vi "Write folder.vi"(8 "error in (no error)":errorcluster, 10 "folder":string="c:\\errorlog", 11 "SimpleErrorLogger in":refnum<class "SimpleErrorLogger.lvclass">) -> (0 "error out":errorcluster, 3 "SimpleErrorLogger out":refnum<class "SimpleErrorLogger.lvclass">)   [LabVIEW 2023, in "SimpleErrorLogger.lvlib" / "SimpleErrorLogger.lvclass"]
uses:
  SimpleErrorLogger.lvclass
  SimpleErrorLogger.lvclass/SimpleErrorLogger.ctl
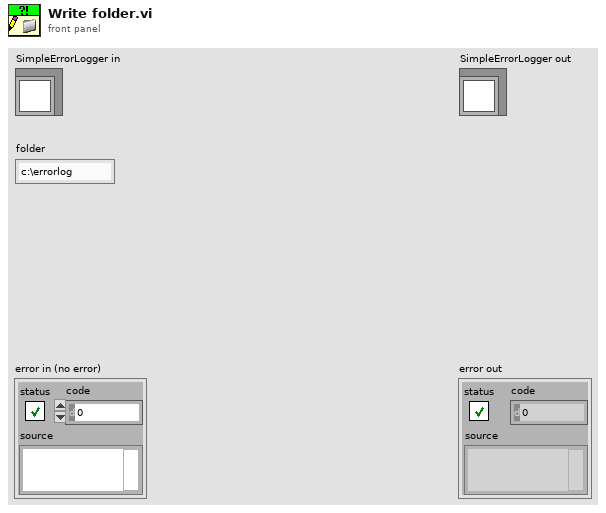
[diagram p1: front panel]
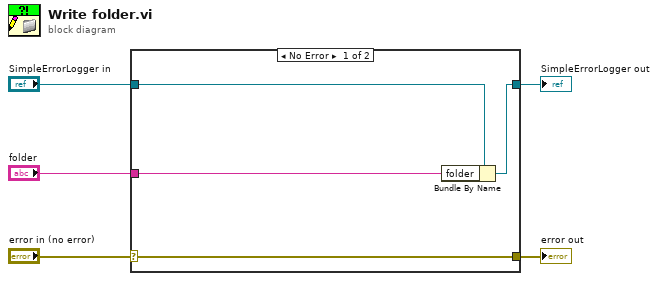
[diagram p0: block diagram]
diagram:
  n1 = case shown="No Error" "error in (no error)" {
    selector: "error in (no error)" -> [w9 w10]
    tunnel: [w9 w10] -> w4
    tunnel: [w7 w11] -> w2
    tunnel: "SimpleErrorLogger in" -> [w8 w11]
    tunnel: "folder" -> [w6 _]
    frame No Error {
      n2 = Bundle By Name(cluster=w8, "folder"=w6) -> (w7:refnum<class "SimpleErrorLogger.lvclass">)
    }
    frame Error {
    }
  }
  "error out" <- w4
  "SimpleErrorLogger out" <- w2
